vi "TimeInterpVariant_GetSample.vi"(4 "Extra":variant, 6 "Interpolate\nReference":refnum<vi>, 9 "TimeStamp":dbl, 11 "TimeInterpVariant":T1) -> (1 "IsPresent":bool, 3 "OutputVariant":variant)   [LabVIEW 2019, in "Trajectory_Library.lvlib"]
doc: "Sample the buffer at the given time.\n\nInputs:\n - TimeInterpVariant -- Input data cluster\n - TimeStamp -- Time at which to sample (seconds)\n\nOutputs\n - OutputPose -- Sampled Variant. This is an exact value if there is a sample in the buffer at this time. Otherwise the value is interpolated. A custom routine will need to be called to extract the custom data from the variant. \n - IsPresent -- Returns TRUE if the buffer contains data as far back as TimeStamp."
uses:
  Trajectory_Library.lvlib
  TypeDef/TIME_INTERPOLATABLE_VARIANT.ctl
  <vilib>/gmath/NI_Gmath.lvlib
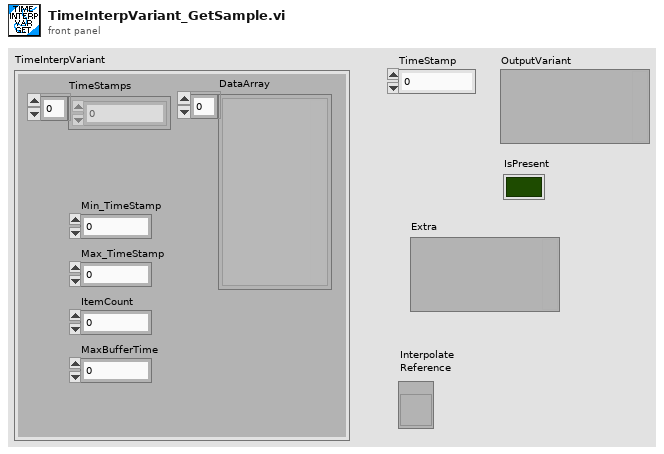
[diagram p1: front panel]
types:
  T1 = typedef "Trajectory_Library.lvlib/TIME_INTERPOLATABLE_VARIANT.ctl" = cluster{"TimeStamps":dbl[], "DataArray":variant[], "Min_TimeStamp":dbl, "Max_TimeStamp":dbl, "ItemCount":i32, "MaxBufferTime":dbl}
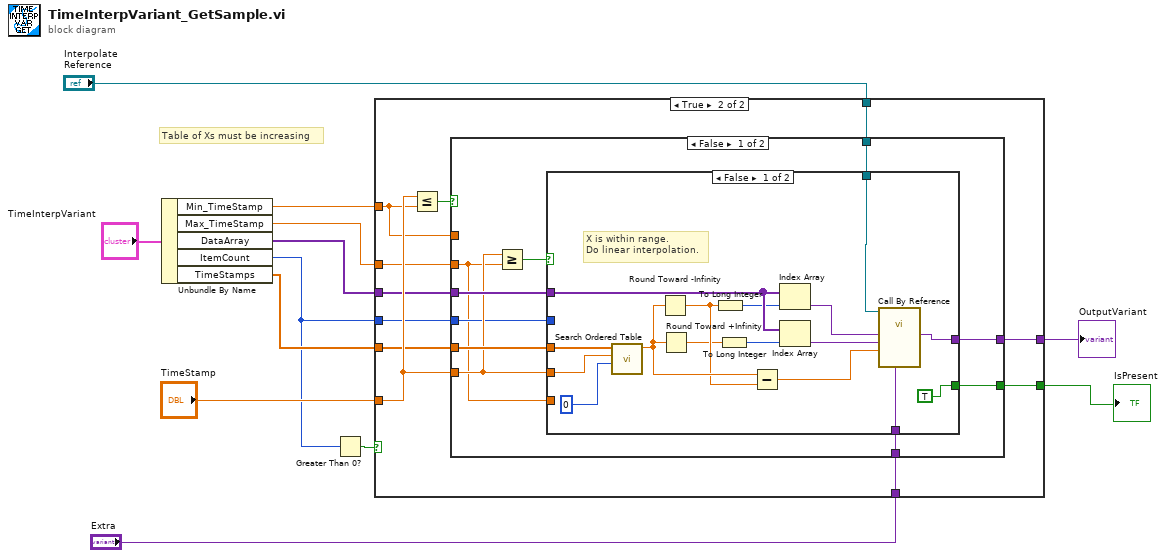
[diagram p0: block diagram]
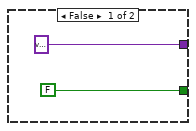
[diagram p2: hidden frame]
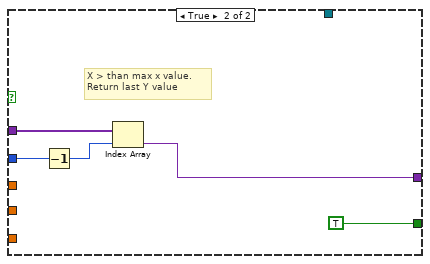
[diagram p3: hidden frame]
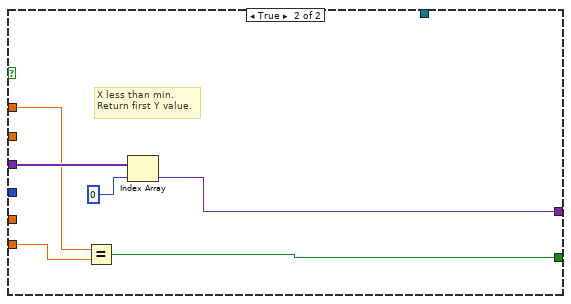
[diagram p4: hidden frame]
diagram:
  # "Table of Xs must be increasing"
  n1 = Unbundle By Name("TimeInterpVariant") -> ("Min_TimeStamp"=w10:dbl, "Max_TimeStamp"=w9:dbl, "DataArray"=w7:variant[], "ItemCount"=w5:i32, "TimeStamps"=w8:dbl[])
  n2 = Greater Than 0?(x=w5) -> (x > 0?=w6:bool)
  n3 = case shown="True" w6 {
    tunnel: "TimeStamp" -> [_ w24]
    tunnel: [variant w23] -> w2
    tunnel: w10 -> [_ w18]
    tunnel: w9 -> [_ w22]
    tunnel: w5 -> [_ w21]
    tunnel: w8 -> [_ w20]
    tunnel: w7 -> [_ w19]
    tunnel: [FALSE w17] -> w4
    tunnel: "Interpolate\nReference" -> [_ w16]
    tunnel: "Extra" -> [_ w15]
    frame False {
    }
    frame True {
      n4 = Less Or Equal?(x=w24, y=w18) -> (x <= y?=w25:bool)
      n5 = case shown="False" w25 {
        tunnel: w19 -> [w34 w62]
        tunnel: [w33 w60] -> w23
        tunnel: w24 -> [w31 w59]
        tunnel: w22 -> [w29 _]
        tunnel: w20 -> [w32 _]
        tunnel: w21 -> [w30 _]
        tunnel: w18 -> [_ w58]
        tunnel: [w28 w57] -> w17
        tunnel: w16 -> [w27 _]
        tunnel: w15 -> [w26 _]
        frame False {
          n6 = Greater Or Equal?(x=w31, y=w29) -> (x >= y?=w35:bool)
          n7 = case shown="False" w35 {
            tunnel: w34 -> [w48 w56]
            tunnel: [w37 w55] -> w33
            tunnel: w32 -> [w50 _]
            tunnel: w31 -> [w49 _]
            tunnel: w30 -> [_ w54]
            tunnel: w29 -> [_ _]
            tunnel: [TRUE TRUE] -> w28
            tunnel: w27 -> [w41 _]
            tunnel: w26 -> [w36 _]
            frame False {
              # "X is within range.  \nDo linear interpolation."
              n8 = call <vilib>:"Search Ordered Table.vi"("starting index"=0, "x value"=w49, "ordered x array"=w50) -> ("fractional index"=w45:dbl)  [unwired: 8 in]
              n9 = Round Toward -Infinity(1:w45) -> (0:w44:dbl)
              n10 = Round Toward +Infinity(x=w45) -> (ceil(x): smallest int >= x=w43:dbl)
              n11 = To Long Integer(number=w44) -> (32bit integer=w47:i32)
              n12 = To Long Integer(number=w43) -> (32bit integer=w46:i32)
              n13 = Subtract(x=w45, y=w44) -> (x-y=w38:dbl)
              n14 = Index Array(array=w48, index=w47) -> (element=w40:variant)
              n15 = Index Array(array=w48, index=w46) -> (element=w39:variant)
              n16 = call-by-ref "?"(reference=w41, "Extra"=w36, "Time Fraction"=w38, "Input 2"=w39, "Input 1"=w40) -> ("Interp Output"=w37:variant)  [unwired: 8 in, 2 out]
            }
            frame True {
              # "X > than max x value.   \nReturn last Y value"
              n17 = Decrement(x=w54) -> (x-1=w53:i32)
              n18 = Index Array(array=w56, index=w53) -> (element=w55:variant)
            }
          }
        }
        frame True {
          # "X less than min.   \nReturn first Y value."
          n19 = Equal?(x=w58, y=w59) -> (x = y?=w57:bool)
          n20 = Index Array(array=w62, index=0) -> (element=w60:variant)
        }
      }
    }
  }
  "OutputVariant" <- w2
  "IsPresent" <- w4
